vi "Graphics-Offset Background Color.vi"(0 "Foreground":u32, 5 "Background":u32, 9 "Fraction":dbl format="%#_13g") -> (4 "Color out":u32)   [LabVIEW 2015]
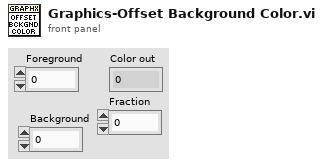
[diagram p1: front panel]
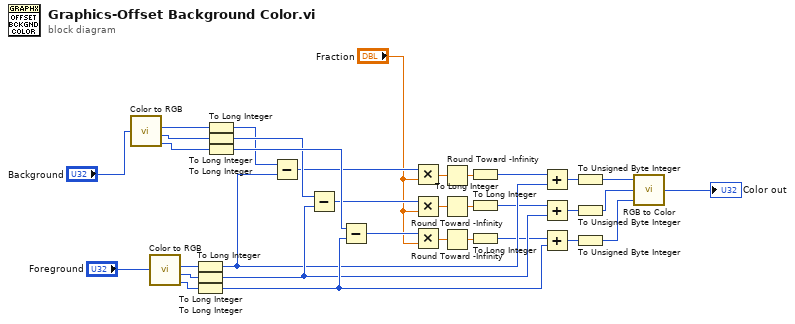
[diagram p0: block diagram]
diagram:
  n1 = call <vilib>:"Color to RGB.vi"("Color"="Background") -> ("R"=w20:u8, "G"=w22:u8, "B"=w23:u8)  [unwired: 1 out]
  n2 = call <vilib>:"Color to RGB.vi"("Color"="Foreground") -> ("R"=w21:u8, "G"=w34:u8, "B"=w24:u8)  [unwired: 1 out]
  n3 = To Long Integer(number=w21) -> (32bit integer=w31:i32)
  n4 = To Long Integer(number=w34) -> (32bit integer=w32:i32)
  n5 = To Long Integer(number=w24) -> (32bit integer=w33:i32)
  n6 = To Long Integer(number=w20) -> (32bit integer=w28:i32)
  n7 = To Long Integer(number=w22) -> (32bit integer=w29:i32)
  n8 = To Long Integer(number=w23) -> (32bit integer=w30:i32)
  n9 = Subtract(x=w28, y=w31) -> (x-y=w25:i32)
  n10 = Subtract(x=w29, y=w32) -> (x-y=w26:i32)
  n11 = Subtract(x=w30, y=w33) -> (x-y=w27:i32)
  n12 = Multiply(x=w25, y="Fraction") -> (x*y=w18:dbl)
  n13 = Multiply(x=w26, y="Fraction") -> (x*y=w16:dbl)
  n14 = Multiply(x=w27, y="Fraction") -> (x*y=w14:dbl)
  n15 = Round Toward -Infinity(1:w18) -> (0:w19:dbl)
  n16 = Round Toward -Infinity(1:w16) -> (0:w17:dbl)
  n17 = Round Toward -Infinity(1:w14) -> (0:w15:dbl)
  n18 = To Long Integer(number=w19) -> (32bit integer=w11:i32)
  n19 = To Long Integer(number=w17) -> (32bit integer=w13:i32)
  n20 = To Long Integer(number=w15) -> (32bit integer=w12:i32)
  n21 = Add(x=w11, y=w31) -> (x+y=w10:i32)
  n22 = Add(x=w13, y=w32) -> (x+y=w9:i32)
  n23 = Add(x=w12, y=w33) -> (x+y=w8:i32)
  n24 = To Unsigned Byte Integer(number=w10) -> (unsigned 8bit integer=w7:u8)
  n25 = To Unsigned Byte Integer(number=w9) -> (unsigned 8bit integer=w6:u8)
  n26 = To Unsigned Byte Integer(number=w8) -> (unsigned 8bit integer=w5:u8)
  n27 = call <vilib>:"RGB to Color.vi"("B"=w5, "G"=w6, "R"=w7) -> ("Color"=→"Color out":u32)
